vi "Message Box.vi"(8 "String 3":string, 9 "String":string) -> (2 "OK respose":bool)   [LabVIEW 2022 SP3]
panel:
  in  "OK Button":bool
  out "String 2":string
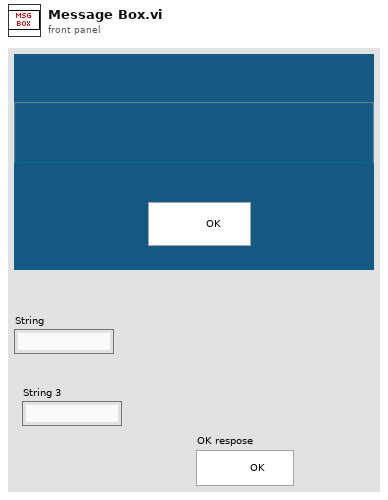
[diagram p1: front panel]
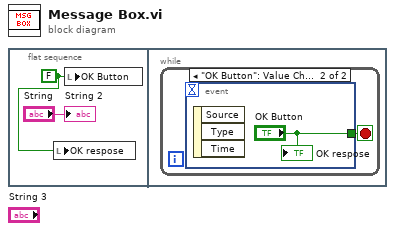
[diagram p0: block diagram]
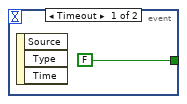
[diagram p2: hidden frame]
diagram:
  n1 = flat-sequence {
    frame #0 {
      w1 = FALSE ("OK Button")
      n2 = local write "OK respose"(w1) -> ()
      n3 = local write "OK Button"(w1) -> ()
      "String 2" <- "String"
    }
    frame #1 {
      n4 = while {
        stop <- w3 stop-if-true
        n5 = event shown="[1] \"OK Button\": Value Change" {
          selector: _ -> [_ _]
          dyn-events: _ -> [_ _]
          timeout: _ -> [_ _]
          tunnel: [FALSE ("OK Button") "OK Button"] -> w3
          event Timeout {
            n6 = event-data() -> ()  [unwired: 1 in, 3 out]
          }
          event "OK Button": Value Change {
            n7 = event-data() -> ()  [unwired: 1 in, 3 out]
            "OK respose" <- "OK Button"
          }
        }
      }
    }
  }
